vi "Assign Parameters to Hardware Dialog.vi"(10 "Hardware Object List":refnum<class "Controller Array.lvclass">, 11 "Parameter to Hardware Map in":refnum<class "Parameter to Hardware Map.lvclass">) -> (3 "Parameter to Hardware Map out":refnum<class "Parameter to Hardware Map.lvclass">)   [LabVIEW 2020]
uses:
  Plugin Servers/Parameter to Hardware Map/Parameter to Hardware Map.lvclass
  Plugin Servers/Controller Array/Controller Array.lvclass
  Plugin Servers/Controller Array/Controller Array.lvclass/Controller Array.ctl
  Plugin Servers/Controller/Generic Plugin.lvclass/Generic Plugin.ctl
  Plugin Servers/Controller/Generic Plugin.lvclass
panel:
  out "Current Hardware":string
  out "Navigate Tree:Get Parent Item":string
  in  "Done":bool
  in  "Parameter Tree":string(tree)
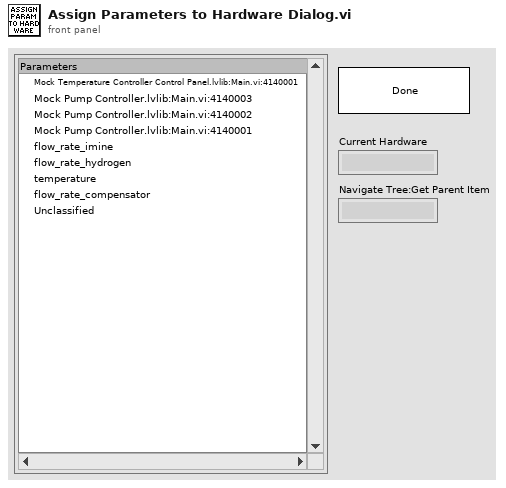
[diagram p1: front panel]
types:
  T1 = cluster{"Left Cell String":string, "Child Text":string[], "Child Tag":string, "Item Indent":i32, "Child Only?":bool, "Glyph Index":i32}
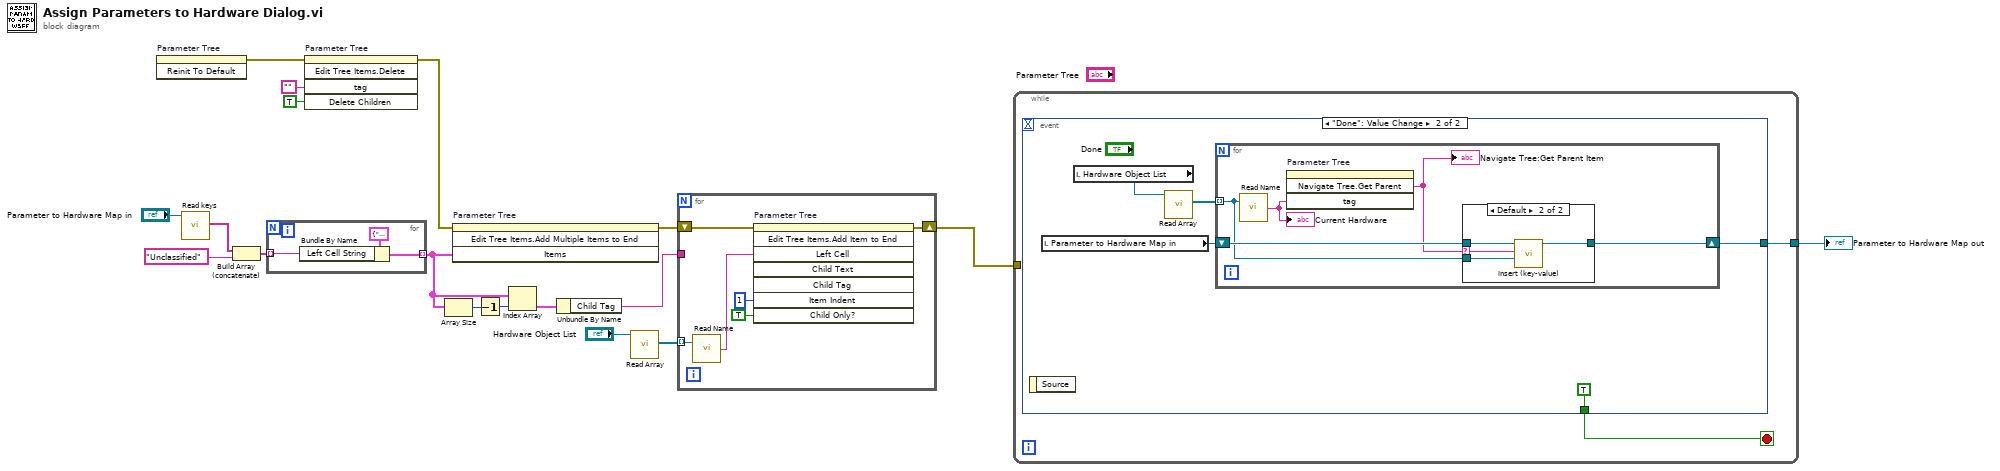
[diagram p0: block diagram]
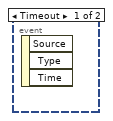
[diagram p2: hidden frame]
diagram:
  n1 = invoke on="Parameter Tree" class="Tree (strict)" method="Reinit To Default"() -> (error out=w8:errorcluster)  [unwired: 3 in, 2 out]
  n2 = call "Read keys.vi"("Parameter to Hardware Map in"="Parameter to Hardware Map in") -> ("Keys"=w11:string[])  [unwired: 8 in, 2 out]
  n3 = Build Array (concatenate)(w11, "Unclassified") -> (w17:string[])
  n4 = for {
    tunnel: w17 -> [w20] mode=indexing
    tunnel: [w19] -> w4 mode=indexing
    n5 = Bundle By Name(cluster=T1 {"Left Cell String"="", "Child Text"=[], "Child Tag"="", "Item Indent"=0, "Child Only?"=FALSE, "Glyph Index"=0} ("Item"), "Left Cell String"=w20) -> (w19:T1)
  }
  n6 = invoke on="Parameter Tree" class="Tree (strict)" method="Edit Tree Items.Delete"(error in=w8, "tag"="", "Delete Children"=TRUE ("Delete Children?")) -> (error out=w13:errorcluster)  [unwired: 2 in, 4 out]
  n7 = Array Size(array=w4) -> (size(s)=w7:i32)
  n8 = invoke on="Parameter Tree" class="Tree (strict)" method="Edit Tree Items.Add Multiple Items to End"(error in=w13, "Items"=w4) -> (error out=w18:errorcluster)  [unwired: 2 in, 3 out]
  n9 = Decrement(x=w7) -> (x-1=w6:i32)
  n10 = Index Array(array=w4, index=w6) -> (element=w5:T1)
  n11 = Unbundle By Name(w5) -> ("Child Tag"=w2:string)
  n12 = call "Read Array.vi"("Controller Array in"="Hardware Object List") -> ("Array"=w1:refnum<class "Generic Plugin.lvclass">[])  [unwired: 8 in, 2 out]
  n13 = for {
    tunnel: w2 -> [_]
    shift-right: [w26] -> w3
    shift-left: w18 -> [w27]
    tunnel: w1 -> [w25] mode=indexing
    n14 = call "Read Name.vi"("controller in"=w25) -> ("Name"=w24:string)  [unwired: 1 in, 2 out]
    n15 = invoke on="Parameter Tree" class="Tree (strict)" method="Edit Tree Items.Add Item to End"(error in=w27, "Left Cell"=w24, "Item Indent"=1 ("New Item Indentation"), "Child Only?"=TRUE) -> (error out=w26:errorcluster)  [unwired: 4 in, 7 out]
  }
  n16 = while {
    tunnel: w3 -> [_]
    tunnel: [w28] -> w9
    stop <- w29 stop-if-true
    n17 = event shown="[1] \"Done\": Value Change" {
      selector: _ -> [_ _]
      dyn-events: _ -> [_ _]
      timeout: _ -> [_ _]
      tunnel: [_ TRUE] -> w29
      tunnel: [_ w30] -> w28
      event Timeout {
        n18 = event-data() -> ()  [unwired: 1 in, 3 out]
      }
      event "Done": Value Change {
        n19 = event-data() -> ()  [unwired: 1 in, 1 out]
        n20 = local read "Parameter to Hardware Map in"() -> (w31:refnum<class "Parameter to Hardware Map.lvclass">)
        n21 = local read "Hardware Object List"() -> (w33:refnum<class "Controller Array.lvclass">)
        n22 = call "Read Array.vi"("Controller Array in"=w33) -> ("Array"=w32:refnum<class "Generic Plugin.lvclass">[])  [unwired: 8 in, 2 out]
        n23 = for {
          tunnel: w32 -> [w37] mode=indexing
          shift-right: [w35] -> w30
          shift-left: w31 -> [w38]
          n24 = call "Read Name.vi"("controller in"=w37) -> ("Name"=w39:string)  [unwired: 1 in, 2 out]
          "Current Hardware" <- w39
          n25 = invoke on="Parameter Tree" class="Tree (strict)" method="Navigate Tree.Get Parent"("tag"=w39) -> ("Navigate Tree:Get Parent"=w36:string)  [unwired: 3 in, 3 out]
          "Navigate Tree:Get Parent Item" <- w36
          n26 = case shown="Default" w36 {
            selector: w36 -> [_ w42]
            tunnel: w38 -> [w40 w44]
            tunnel: w37 -> [_ w43]
            tunnel: [w40 w41] -> w35
            frame "Unclassified" {
            }
            frame Default {
              n27 = call "Insert (key-value).vi"("Value"=w43, "Key"=w42, "Parameter to Hardware Map in"=w44) -> ("Parameter to Hardware Map out"=w41:refnum<class "Parameter to Hardware Map.lvclass">)  [unwired: 7 in, 1 out]
            }
          }
        }
      }
    }
  }
  "Parameter to Hardware Map out" <- w9
